vi "IMA Wait for DC Start.vi"(0 "WFDC External Sync":refnum<notifier>, 11 "Error":errorcluster) -> (4 "WFDC External Sync (Dup)":refnum<notifier>, 15 "Error Out":errorcluster)   [LabVIEW 2016]
uses:
  Wide Field Drift Correction/WFDC Controls/WFDC External Sync.ctl
  Wide Field Drift Correction/WFDC Controls/WFDC Cycle Pause.ctl
  Wide Field Drift Correction/WFDC Controls/WFDC Status.ctl
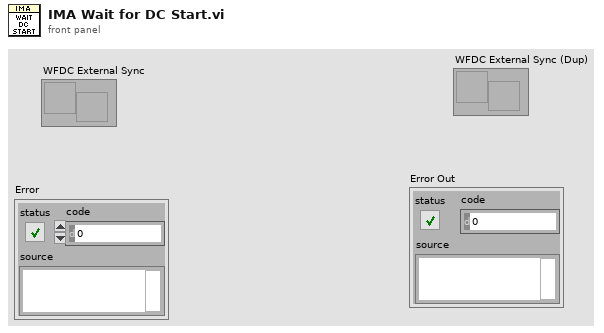
[diagram p1: front panel]
types:
  T1 = typedef "WFDC Status.ctl" = enum16{"Idle", "Busy", "DC Active", "Error"}
  T2 = typedef "WFDC External Sync.ctl" = cluster{"Cycle Sync":T3, "Z Offset":dbl, "WFDC Status":T1}
  T3 = typedef "WFDC Cycle Pause.ctl" = enum16{"Pause Requested", "Paused", "Resume Requested", "Resumed"}
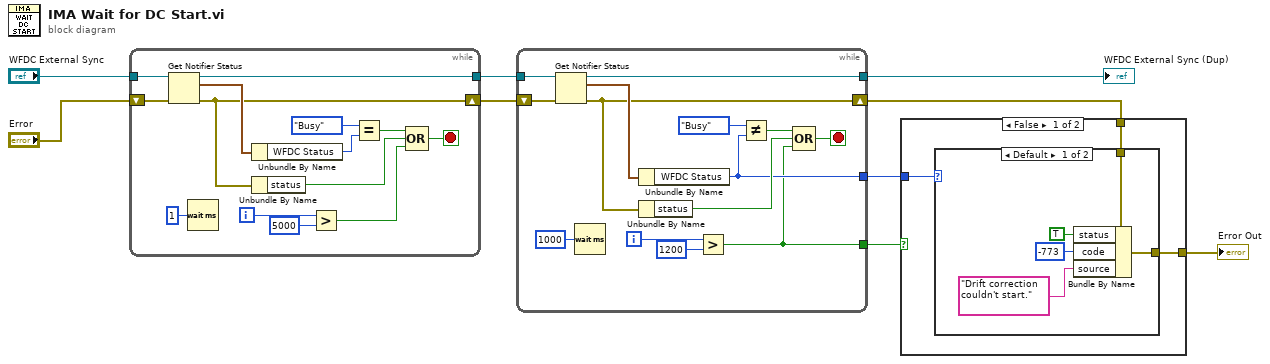
[diagram p0: block diagram]
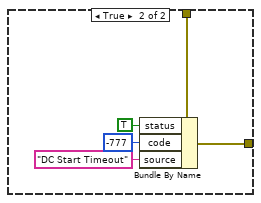
[diagram p3: hidden frame]
diagram:
  n1 = while {
    tunnel: "WFDC External Sync" -> [w22]
    tunnel: [w20] -> w6
    shift-right: [w16] -> w5
    shift-left: "Error" -> [w19]
    i -> [w15]
    stop <- w11 stop-if-true
    n2 = Get Notifier Status(notifier=w22, error in (no error)=w19) -> (notifier out=w20:refnum<notifier>, current notification=w23:T2, error out=w16:errorcluster)  [unwired: 2 out]
    n3 = Wait (ms)(milliseconds to wait=u32 1) -> ()  [unwired: 1 out]
    n4 = Unbundle By Name(w23) -> ("WFDC Status"=w17:T1)
    n5 = Unbundle By Name(w16) -> ("status"=w12:bool)
    n6 = Greater?(x=w15, y=5000) -> (0:w10:bool)
    n7 = Equal?(x=WFDC_Status."Busy", y=w17) -> (x = y?=w13:bool)
    n8 = Compound Arithmetic op=OR(w13, w12, w10) -> (w11:bool)
  }
  n9 = while {
    tunnel: w6 -> [w36]
    tunnel: [w34] -> w9
    shift-right: [w31] -> w3
    shift-left: w5 -> [w33]
    tunnel: [w25] -> w2
    tunnel: [w24] -> w4
    i -> [w30]
    stop <- w26 stop-if-true
    n10 = Get Notifier Status(notifier=w36, error in (no error)=w33) -> (notifier out=w34:refnum<notifier>, current notification=w37:T2, error out=w31:errorcluster)  [unwired: 2 out]
    n11 = Wait (ms)(milliseconds to wait=u32 1000) -> ()  [unwired: 1 out]
    n12 = Unbundle By Name(w37) -> ("WFDC Status"=w25:T1)
    n13 = Unbundle By Name(w31) -> ("status"=w27:bool)
    n14 = Greater?(x=w30, y=1200) -> (0:w24:bool)
    n15 = Not Equal?(x=WFDC_Status."Busy", y=w25) -> (x != y?=w28:bool)
    n16 = Compound Arithmetic op=OR(w28, w27, w24) -> (w26:bool)
  }
  "WFDC External Sync (Dup)" <- w9
  n17 = case shown="False" w4 {
    tunnel: w3 -> [w38 w47]
    tunnel: [w39 w48] -> w1
    tunnel: w2 -> [w40 _]
    frame False {
      n18 = case shown="Default" w40 {
        tunnel: [w41 w46] -> w39
        tunnel: w38 -> [w45 w46]
        frame Default {
          n19 = Bundle By Name(cluster=w45, "status"=TRUE, "code"=-773, "source"="Drift correction couldn't start.") -> (w41:errorcluster)
        }
        frame "DC Active" {
        }
      }
    }
    frame True {
      n20 = Bundle By Name(cluster=w47, "status"=TRUE, "code"=-777, "source"="DC Start Timeout") -> (w48:errorcluster)
    }
  }
  "Error Out" <- w1
